vi "ConvEncode.vi"(8 "error in (no error)":errorcluster, 10 "Encode Parameter":T1={"constraint length (K)"=3, "initial state"=0, "Encode factor"=0} {"initial state" format="%.0x"}, 11 "Input Bits":i8[](array[numeric])) -> (0 "error out":errorcluster, 3 "output bit stream":i8[](array[numeric]))   [LabVIEW 2014]
uses:
  <vilib>/addons/Modulation/Digital/Channel Coding/MT Convolutional Encoder (Rate).vi
  <vilib>/addons/Modulation/Digital/Support/Common/Validators/mod_Validate Bit Stream.vi
  <vilib>/addons/Modulation/Digital/Channel Coding/Convolutional codes/mod_Convolutional encoder.vi
  <vilib>/addons/Modulation/Analog/support/mod_Set Error Source.vi
  <vilib>/addons/Modulation/Digital/Channel Coding/Convolutional codes/subVIs/mod_Generate encoder tap connections.vi
  <vilib>/addons/Modulation/Digital/Channel Coding/Convolutional codes/subVIs/mod_Perform convolutional encoding.vi
  <vilib>/addons/Modulation/Digital/Channel Coding/Block codes/subVIs/mod_Buffer block code info (I8).vi
  <vilib>/addons/Modulation/Digital/Channel Coding/Convolutional codes/subVIs/mod_Generate valid reset (convolutional, I8).vi
  <vilib>/addons/Modulation/Digital/Channel Coding/Convolutional codes/subVIs/mod_Select known generator matrix.vi
  <vilib>/addons/Modulation/Digital/Support/Common/Validators/mod_Validate Convolutional Encoder prms.vi
  <vilib>/addons/Modulation/niDMT.lvlib
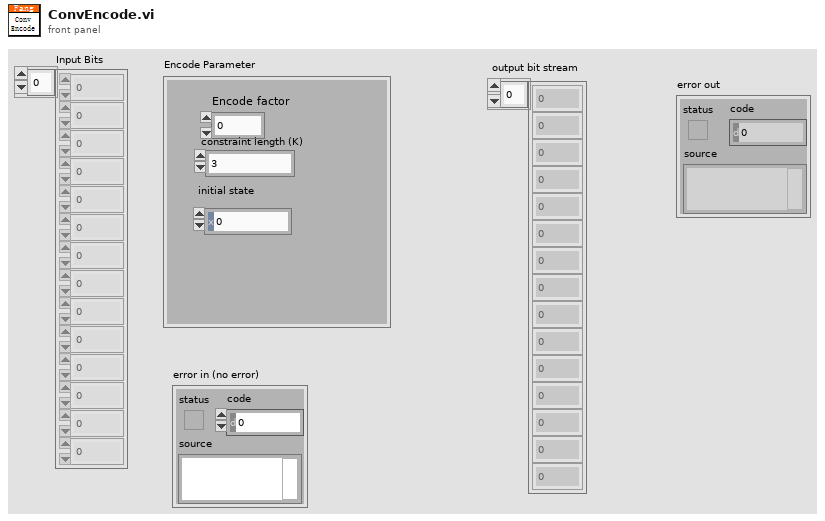
[diagram p1: front panel]
types:
  T1 = cluster{"constraint length (K)":i32, "initial state":u32, "Encode factor":i32}
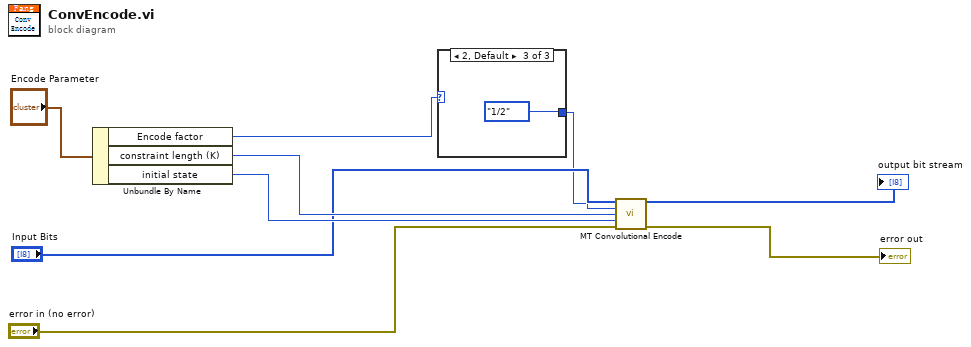
[diagram p0: block diagram]
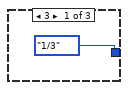
[diagram p2: hidden frame]
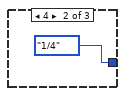
[diagram p3: hidden frame]
diagram:
  n1 = Unbundle By Name("Encode Parameter") -> ("Encode factor"=w2:i32, "constraint length (K)"=w8:i32, "initial state"=w7:u32)
  n2 = case shown="2, Default" w2 {
    tunnel: [enum16{"1/2", "1/3", "1/4", "2/3", "3/4"}."1/3" ("rate (k/n)") enum16{"1/2", "1/3", "1/4", "2/3", "3/4"}."1/4" ("rate (k/n)") enum16{"1/2", "1/3", "1/4", "2/3", "3/4"}."1/2" ("rate (k/n)")] -> w1
    frame 3 {
    }
    frame 4 {
    }
    frame 2, Default {
    }
  }
  n3 = call-poly <vilib>:"MT Convolutional Encode.vi"("input bit stream"="Input Bits", "rate (k/n)"=w1, "constraint length (K)"=w8, "initial state"=w7, "error in (no error)"="error in (no error)") -> ("output bit stream"=→"output bit stream":i8[], "error out"=→"error out":errorcluster)  [unwired: 8 in, 1 out]
